vi "0-WaypointInput.vi"() -> ()   [LabVIEW 2011]
panel:
  out "# of Waypts":i32
  in  "stop":bool
  in  "Save Waypoints\nand PoI":bool
  in  "Delete Last Waypoint":bool
  out "Mission Map":T1(plugin-control)
  in  "Map Path (relative)":path=path "locations/LPB Pool.png"
  in  "Save Image":bool
  in  "MDF (Mission Definition File) path (leave blank for nothing)":path
  # "Usage"
  # "Map (required) and MDF (optional) are loaded on start\nClick on map to add waypoints\nClick the appropriate buttons to load/save MDFs."
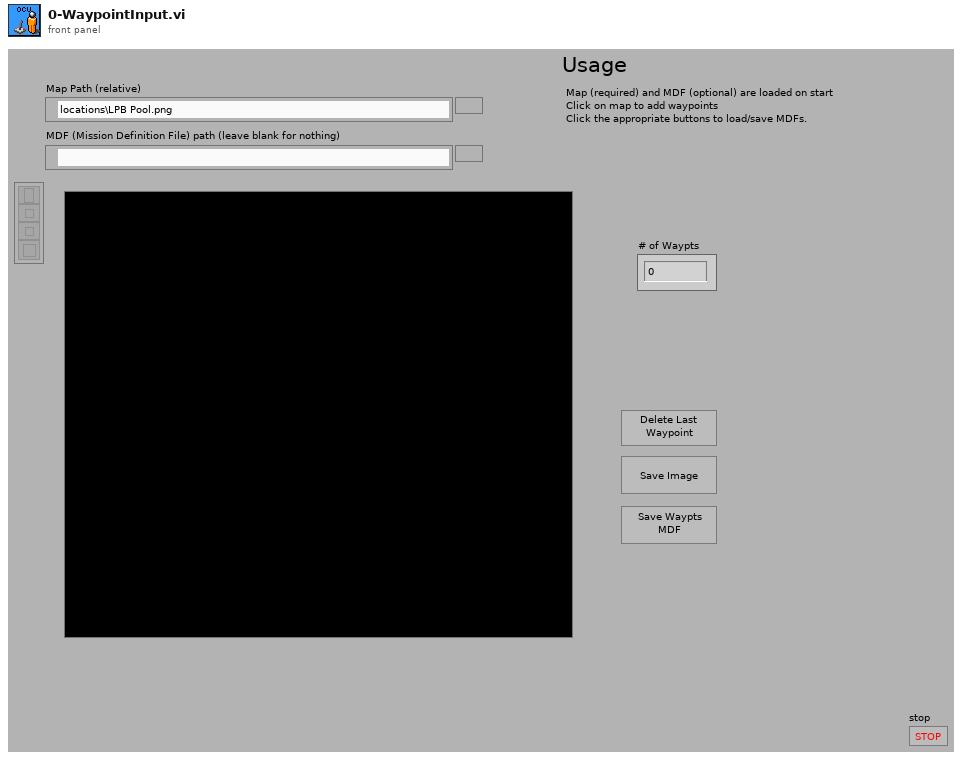
[diagram p1: front panel]
types:
  T1 = typedef "IMAQ Image.ctl" = refnum<image>
  T2 = typedef "Waypoints List.ctl" = T3[]
  T3 = typedef "ocuWaypoint.ctl" = cluster{"Point Type":T4, "Dist/Time":dbl, "UTM Location":T5}
  T4 = typedef "waypointTypes.ctl" = enum16{"Drive", "Round Port", "Round Starboard", "Stay"}
  T5 = typedef "UTM Location.ctl" = cluster{"UTM Zone":dbl, "Hemisphere":enum16{"North", "South"}, "East":dbl, "North":dbl}
  T6 = typedef "0-Image Descriptor.ctl" = cluster{"Upper-Left Corner Coordinates":T5, "Meters/Pixel":dbl}
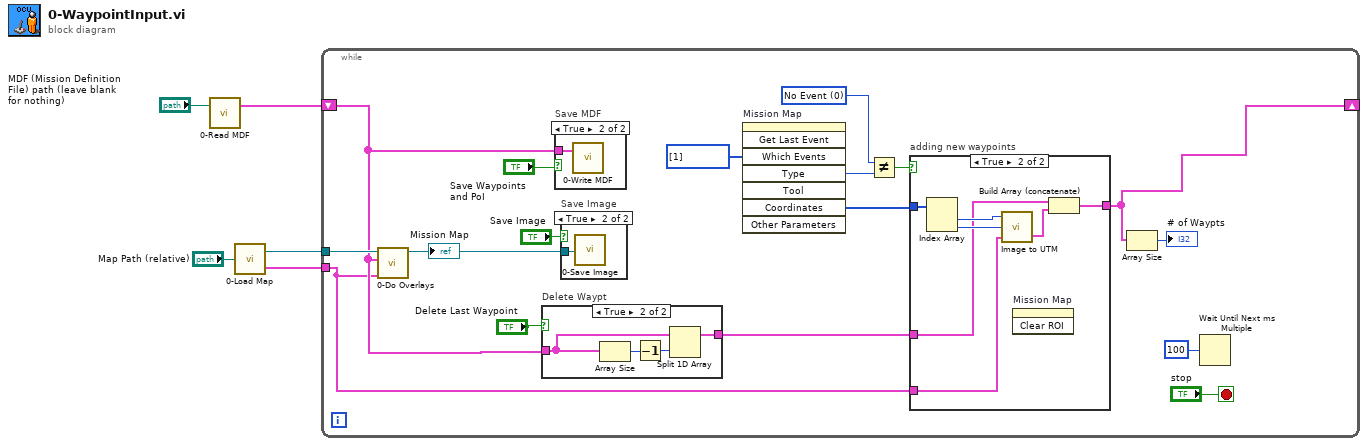
[diagram p0: block diagram]
diagram:
  n1 = call "0-Read MDF.vi"("MDF file"="MDF (Mission Definition File) path (leave blank for nothing)") -> ("Waypoints List"=w1:T2)  [unwired: 2 in]
  n2 = call "0-Load Map.vi"("Image Path"="Map Path (relative)") -> ("Image Out"=w4:T1, "Image Descriptor"=w3:T6)
  n3 = while {
    tunnel: w4 -> [w22]
    tunnel: w3 -> [w6]
    shift-right: [w7] -> _
    shift-left: w1 -> [w8]
    stop <- "stop" stop-if-true
    w18 = 0 items=["No Event"=0, "Click Event"=1, "Draw Event"=2, "Size Event"=4, "Scroll Event"=5, "Double Click Event"=8] ("Type")
    n4 = call "0-Do Overlays.vi"("Image Descriptor"=w6, "Waypoints List"=w8, "Image in"=w22) -> ("Image out"=w11:T1)  [unwired: 8 in]
    "Mission Map" <- w11
    n5 = case "Delete Waypt" shown="True" "Delete Last Waypoint" {
      tunnel: [w25 w26] -> w14
      tunnel: w8 -> [w25 w29]
      frame False {
      }
      frame True {
        n6 = Array Size(array=w29) -> (size(s)=w28:i32)
        n7 = Decrement(x=w28) -> (x-1=w27:i32)
        n8 = Split 1D Array(array=w29, index=w27) -> (first subarray=w26:T2)  [unwired: 1 out]
      }
    }
    n9 = case "Save MDF" shown="True" "Save Waypoints\nand PoI" {
      tunnel: w8 -> [_ w23]
      frame False {
      }
      frame True {
        n10 = call "0-Write MDF.vi"("Waypoints List"=w23) -> ()  [unwired: 3 in]
      }
    }
    n11 = case "Save Image" shown="True" "Save Image" {
      tunnel: w11 -> [_ w24]
      frame False {
      }
      frame True {
        n12 = call "0-Save Image.vi"("Image in"=w24) -> ()  [unwired: 10 in, 1 out]
      }
    }
    n13 = invoke on="Mission Map" class="ImageControl" method="Get Last Event"("Which Events"=i32[] [1]) -> ("Type"=w19:i32, "Coordinates"=w16:i32[])  [unwired: 7 in, 6 out]
    n14 = Not Equal?(x=w18, y=w19) -> (x != y?=w21:bool)
    n15 = case "adding new waypoints" shown="True" w21 {
      tunnel: w14 -> [w30 w32]
      tunnel: [w30 w33] -> w7
      tunnel: w16 -> [_ w37]
      tunnel: w6 -> [_ w34]
      frame False {
      }
      frame True {
        n16 = Index Array(array=w37) -> (element #1=w36:i32, element #2=w35:i32)  [unwired: 2 in]
        n17 = call "Image to UTM.vi"("Image Descriptor"=w34, "Y"=w35, "X"=w36) -> ("Waypoint"=w31:T3)  [unwired: 1 out]
        n18 = invoke on="Mission Map" class="ImageControl" method="Clear ROI"() -> ()  [unwired: 3 in, 3 out]
        n19 = Build Array (concatenate)(w32, w31) -> (w33:T2)
      }
    }
    n20 = Array Size(array=w7) -> (size(s)=→"# of Waypts":i32)
    n21 = Wait Until Next ms Multiple(millisecond multiple=u32 100 ("milliseconds to wait")) -> ()  [unwired: 1 out]
  }
